vi "ConfigureROI.vi"(0 "object in":refnum<class "Hamamatsu.lvclass">, 2 "Sub Region":T3, 5 "error in (no error)":errorcluster) -> (14 "object out":refnum<class "Hamamatsu.lvclass">, 16 "SubRegionLimits":T1 {"V Size"."Value" min=0 max=0 step=4; "H Size"."Value" min=0 max=0 step=4; "V Offset"."Value" min=0 max=0 step=4; "H Offset"."Value" min=0 max=0 step=4}, 19 "error out":errorcluster)   [LabVIEW 2023, in "Hamamatsu.lvclass"]
uses:
  Hamamatsu.lvclass
  SubRegion.ctl
  SubRegionLimits.ctl
  <vilib>/Utility/miscctls.llb/LVMinMaxIncTypeDef.ctl
  Hamamatsu.lvclass/Hamamatsu.ctl
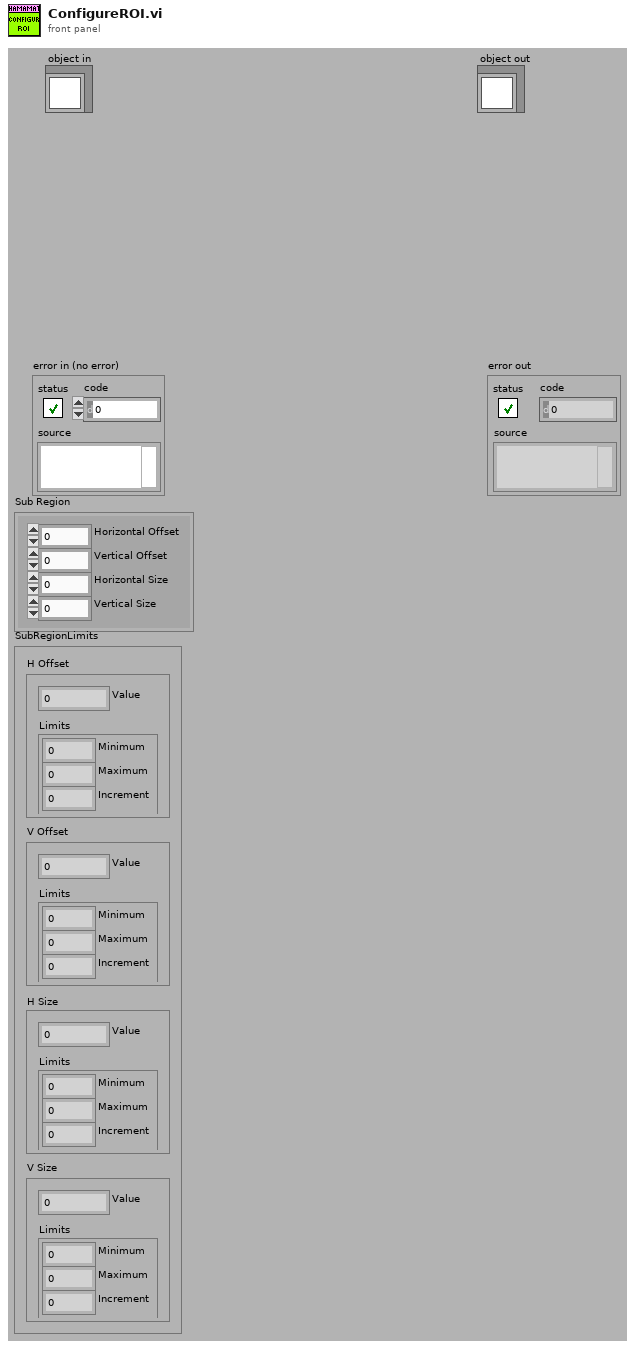
[diagram p1: front panel]
types:
  T1 = typedef "Hamamatsu.lvclass/SubRegionLimits.ctl" = cluster{"H Offset":cluster{"Value":i32, "Limits":T2}, "V Offset":cluster{"Value":i32, "Limits":T2}, "H Size":cluster{"Value":i32, "Limits":T2}, "V Size":cluster{"Value":i32, "Limits":T2}}
  T2 = typedef "LVMinMaxIncTypeDef.ctl" = cluster{"Minimum":dbl, "Maximum":dbl, "Increment":dbl}
  T3 = typedef "Hamamatsu.lvclass/SubRegion.ctl" = cluster{"Horizontal Offset":i32, "Vertical Offset":i32, "Horizontal Size":i32, "Vertical Size":i32}
  T4 = cluster{"H Offset":cluster{"Value":i32, "Limits":T2}, "V Offset":cluster{"Value":i32, "Limits":T2}, "H Size":cluster{"Value":i32, "Limits":T2}, "V Size":cluster{"Value":i32, "Limits":T2}}
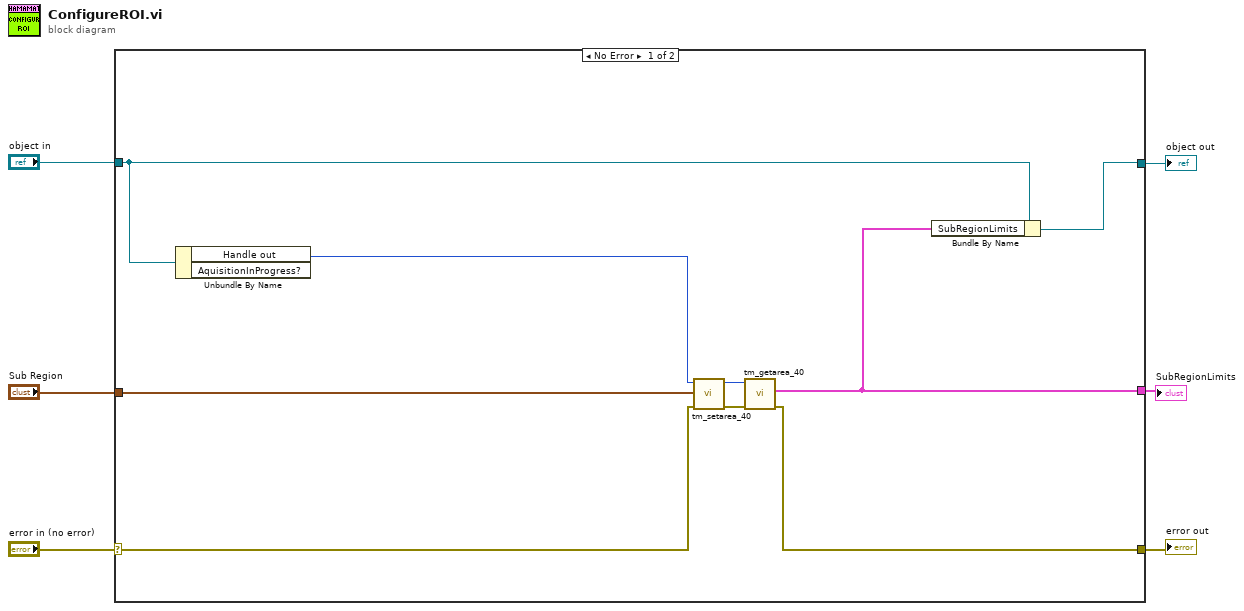
[diagram p0: block diagram]
diagram:
  n1 = case shown="No Error" "error in (no error)" {
    selector: "error in (no error)" -> [w12 w17]
    tunnel: [w10 w17] -> w5
    tunnel: [w8 w16] -> w3
    tunnel: "object in" -> [w7 w16]
    tunnel: "Sub Region" -> [w11 _]
    tunnel: [w9 _] -> w1
    frame No Error {
      n2 = Unbundle By Name(w7) -> ("Handle out"=w15:u32)  [unwired: 1 out]
      n3 = call <userlib>:"tm_setarea_40.vi"("error in (no error)"=w12, "Sub Region"=w11, "Handle in"=w15) -> ("error out"=w13:errorcluster, "Handle out"=w14:u32)  [unwired: 7 in]
      n4 = call <userlib>:"tm_getarea_40.vi"("error in (no error)"=w13, "Handle in"=w14) -> ("error out"=w10:errorcluster, "Sub Region"=w9:T4)  [unwired: 7 in, 1 out]
      n5 = Bundle By Name(cluster=w7, "SubRegionLimits"=w9) -> (w8:refnum<class "Hamamatsu.lvclass">)
    }
    frame Error {
    }
  }
  "error out" <- w5
  "object out" <- w3
  "SubRegionLimits" <- w1
